vi "Check spreadsheet col for dups.vi"(8 "error in (no error)":errorcluster, 10 "col":i32, 11 "Sorted Spreadsheet":string[][](array[string])) -> (0 "error out":errorcluster, 3 "Got dups?":bool)   [LabVIEW 2013]
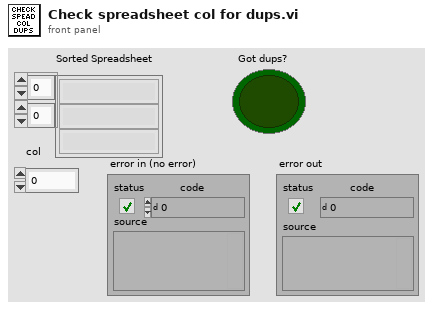
[diagram p1: front panel]
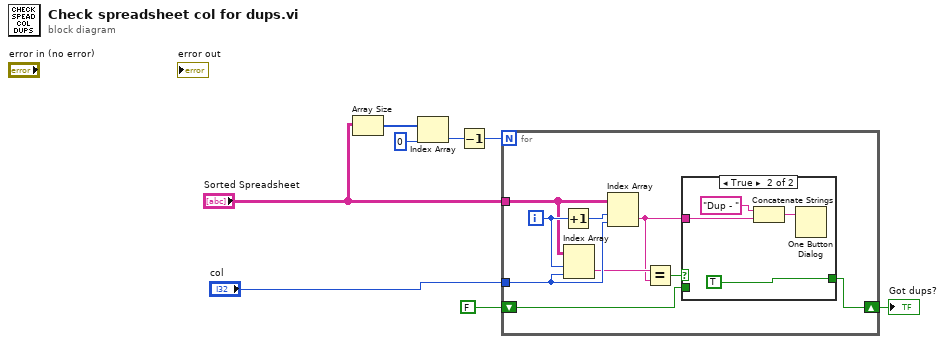
[diagram p0: block diagram]
diagram:
  n1 = Array Size(array="Sorted Spreadsheet") -> (size(s)=w2:i32[])
  n2 = Index Array(array=w2, index=0) -> (element=w4:i32)
  n3 = Decrement(x=w4) -> (x-1=w5:i32)
  n4 = for {
    N: w5 -> [_]
    tunnel: "Sorted Spreadsheet" -> [w13]
    tunnel: "col" -> [w15]
    shift-right: [w9] -> w8
    shift-left: FALSE -> [w10]
    i -> [w17]
    n5 = Increment(x=w17) -> (x+1=w16:i32)
    n6 = Index Array(array=w13, index (row)=w17, index (col)=w15) -> (element=w14:string)
    n7 = Index Array(array=w13, index (row)=w16, index (col)=w15) -> (element=w12:string)
    n8 = Equal?(x=w14, y=w12) -> (x = y?=w11:bool)
    n9 = case shown="True" w11 {
      tunnel: w12 -> [_ w21]
      tunnel: w10 -> [w18 _]
      tunnel: [w18 TRUE ("y")] -> w9
      frame False {
      }
      frame True {
        n10 = Concatenate Strings("Dup - " ("string"), w21) -> (w20:string)
        n11 = One Button Dialog(message=w20) -> ()  [unwired: 1 in, 1 out]
      }
    }
  }
  "Got dups?" <- w8
